vi "Crab+Snake.vi"(0 "RobotDriveDevRef":T1={"DevStatus"={"status"=FALSE, "code"=0, "source"=""}, "Motors[]"=[], "Square Inputs"=FALSE, "Max Output"=1.0, "Isochronous"=FALSE}, 1 "RobotPivotDevRef":T1={"DevStatus"={"status"=FALSE, "code"=0, "source"=""}, "Motors[]"=[], "Square Inputs"=FALSE, "Max Output"=1.0, "Isochronous"=FALSE}, 2 "Joystick 1 X":dbl, 3 "Joystick 1 Y":dbl, 4 "Joystick 2 X":dbl, 5 "error in (no error)":errorcluster, 7 "Rear Left Current Pivot Angle":dbl, 9 "Rear Right Current Pivot Angle":dbl, 11 "Front Left Current Pivot Angle":dbl, 13 "Front Right Current Pivot Angle":dbl) -> (14 "RobotDriveDevRef Out":T1={"DevStatus"={"status"=FALSE, "code"=0, "source"=""}, "Motors[]"=[], "Square Inputs"=FALSE, "Max Output"=1.0, "Isochronous"=FALSE}, 15 "RobotPivotDevRef Out":T1={"DevStatus"={"status"=FALSE, "code"=0, "source"=""}, "Motors[]"=[], "Square Inputs"=FALSE, "Max Output"=1.0, "Isochronous"=FALSE}, 19 "error out":errorcluster)   [LabVIEW 2011, in "Pivot Drive.lvlib"]
doc: "A convience VI. This implments the pivot drive VI in such a way that not as many inputs or calculations are required. Crab changes the robot dirrection without changing the orientation. Snake changes the orientation. Together the robot can move in any dirrection while changing its orientation."
uses:
  Pivot Drive.lvlib
  <vilib>/Rock Robotics/WPI/RobotDrive/WPI_RobotDriveDevRef.ctl
  <vilib>/Rock Robotics/WPI/MotorControl/WPI_MotorControlDeviceRef.ctl
  <vilib>/Rock Robotics/SystemInterfaces/Typedef/FPGA_TypedefDigitalModule.ctl
  <vilib>/Rock Robotics/SystemInterfaces/DIO/FPGA_DIOPWMChannel.ctl
  <vilib>/Rock Robotics/WPI/PWM/WPI_PWMDeadband.ctl
  <vilib>/Rock Robotics/WPI/CAN/Jaguar/SubVIs/WPI_CANJaguar_ControlMode.ctl
  <vilib>/Rock Robotics/WPI/PWM/WPI_PWMTransform_ConPane.ctl
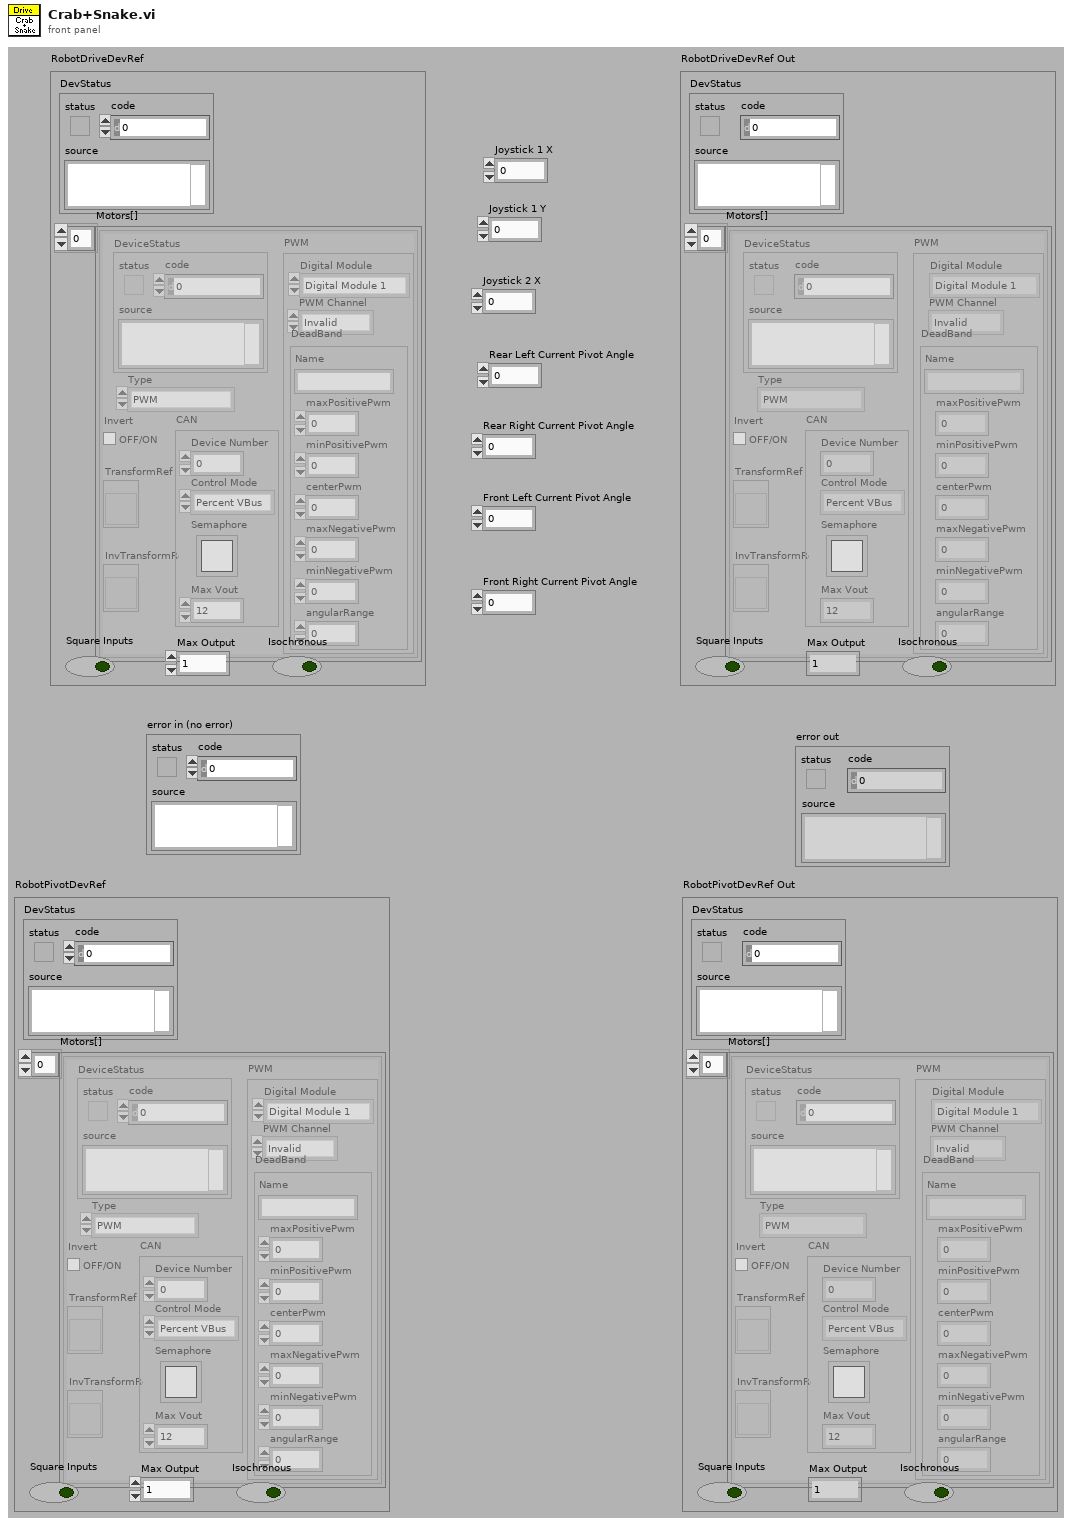
[diagram p1: front panel]
types:
  T1 = typedef "WPI_RobotDriveDevRef.ctl" = cluster{"DevStatus":errorcluster, "Motors[]":T2[], "Square Inputs":bool, "Max Output":dbl, "Isochronous":bool}
  T2 = typedef "WPI_MotorControlDeviceRef.ctl" = cluster{"DeviceStatus":errorcluster, "Type":enum16{"PWM", "CAN"}, "PWM":cluster{"Digital Module":T3, "PWM Channel":T4, "DeadBand":T5}, "CAN":cluster{"Device Number":u8, "Control Mode":T6, "Semaphore":T7, "Max Vout":dbl}, "Invert":bool, "TransformRef":T8, "InvTransformRef":T8}
  T3 = typedef "FPGA_TypedefDigitalModule.ctl" = enum16{"Digital Module 1", "Digital Module 2"}
  T4 = typedef "FPGA_DIOPWMChannel.ctl" = enum8{"PWM 1", "PWM 2", "PWM 3", "PWM 4", "PWM 5", "PWM 6", "PWM 7", "PWM 8", "PWM 9", "PWM 10", "Invalid"}
  T5 = typedef "WPI_PWMDeadband.ctl" = cluster{"Name":string, "maxPositivePwm":i32, "minPositivePwm":i32, "centerPwm":i32, "maxNegativePwm":i32, "minNegativePwm":i32, "angularRange":u16}
  T6 = typedef "WPI_CANJaguar_ControlMode.ctl" = enum8{"Percent VBus", "Current", "Speed", "Position", "Voltage"}
  T7 = typedef "Semaphore RefNum" = refnum<k1>
  T8 = typedef "WPI_PWMTransform_ConPane.ctl" = refnum<vi>
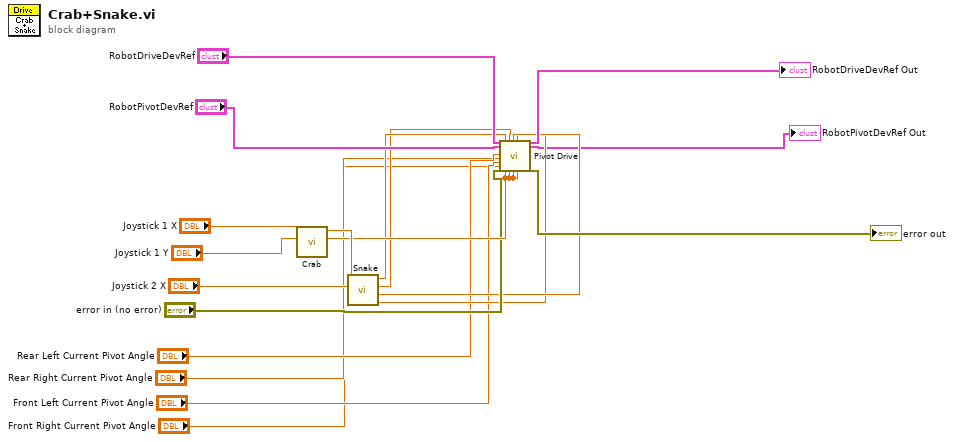
[diagram p0: block diagram]
diagram:
  n1 = call "Crab.vi"("J1 Y"="Joystick 1 Y", "J1 X"="Joystick 1 X") -> ("Magnitude"=w13:dbl, "Joystick Degree"=w16:dbl)  [unwired: 8 out]
  n2 = call "Snake.vi"("Snake"="Joystick 2 X", "Crab Degree"=w16) -> ("FR"=w6:dbl, "FL"=w7:dbl, "RR"=w8:dbl, "RL"=w9:dbl)  [unwired: 6 out]
  n3 = call "Pivot Drive.vi"("RobotDriveDevRef"="RobotDriveDevRef", "RobotPivotDevRef"="RobotPivotDevRef", "Rear Left Current Pivot Angle"="Rear Left Current Pivot Angle", "Rear Right Current Pivot Angle"="Rear Right Current Pivot Angle", "Front Left Current Pivot Angle"="Front Left Current Pivot Angle", "Front Right Current Pivot Angle"="Front Right Current Pivot Angle", "error in (no error)"="error in (no error)", "Rear Left Wanted Pivot Angle"=w9, "Rear Left Speed"=w13, "Rear Right Wanted Pivot Angle"=w8, "Rear Right Speed"=w13, "Front Left Wanted Pivot Angle"=w7, "Front Left Speed"=w13, "Front Right Wanted Pivot Angle"=w6, "Front Right Speed"=w13) -> ("RobotDriveDevRef Out"=→"RobotDriveDevRef Out":T1, "RobotPivotDevRef Out"=→"RobotPivotDevRef Out":T1, "error out"=→"error out":errorcluster)  [unwired: 2 in, 8 out]
